vi "Fetch Measurement.vi"   [LabVIEW 2016, in "Yokogawa WT300 Series.lvlib"]
doc: "Queries the waveform measurement value.\n\nNote:\n(1) If the measurement is not possible, \"NAN (Not A Number)\" is returned."
uses:
  Yokogawa WT300 Series.lvlib
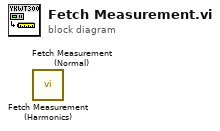
[diagram p0: block diagram]
diagram:
  n1 = call "Fetch Measurement (Harmonics).vi"() -> ()  [unwired: 8 in, 4 out]
  n2 = call "Fetch Measurement (Normal).vi"() -> ()  [unwired: 8 in, 4 out]
